vi "Meas Process Config Panel.vi"(8 "error in (no error)":errorcluster, 11 "session in":T1={"adc"={"niScope"={"channel cfg"=[], "sessions"=[], "multi cards"=FALSE, "channels"=0, "type"=enum."n/a", "memory [B/chn]"=0, "ext. clock [Hz]"=0.0, "samples count"=0, "use streaming"=FALSE, "proc setup"={"packet size [smpl]"=0, "current timeout [s]"=0.0, "blk2blk timeout [s]"=0.0, "event time"=timestamp(0 s since 1904-01-01), "temp sampl T [s]"=0.0, "data queue"=refnum, "stop notifier"=refnum, "proc ref"=refnum}, "sample width [B]"=0, "ranges [V]"=[], "trigger setup"={"coupling"=1, "level [V]"=0.0, "slope"=0, "mode"=enum."Immediate"}, "fs [Hz]"=0.0, "bitres [bit]"=0}, "3458A"={"channels"=[], "sync unit"={"VISA"="", "type"=enum."Picotest U6200A"}, "awg unit"={"type"=enum."Agilent 331xxA to 332xxA", "VISA"="", "enable 10MHz ref"=FALSE}, "sync mode"=enum."MASTER-SLAVE, MASTER clocked by TIMER", "streaming mode"=FALSE, "idn mode"=enum."Auto", "sampling mode"=enum."DCV", "Ts [s]"=0.0, "sample memory [B]"=0, "proc setup"={"channel id"=0, "packet size [smpl]"=0, "current timeout [s]"=0.0, "blk2blk timeout [s]"=0.0, "event time"=timestamp(0 s since 1904-01-01), "stop notifier"=refnum, "data queues"=[], "proc refs"=[], "bus semaphore"=refnum}, "sample size [B]"=0, "sample count"=0, "aux data"={"channel id"=0, "valid?"=[], "gain [V]"=[], "timestamp [s]"=[], "Ts [s]"=0.0, "abs timestamp"=timestamp(0 s since 1904-01-01), "t [deg C]"=[]}, "ranges [V]"=[], "aperture [s]"=0.0, "LEVEL trigger"={"edge"=enum."POS", "level [V]"=0.0, "coupling"=enum."DC"}, "trigger mode"=enum."AUTO", "measure temp.?"=FALSE, "disp mesages"=[], "shared bus?"=FALSE, "disable display?"=FALSE, "aper mode"=enum."Manual", "aper rules"=[]}, "dsdll"={"dsdll"={"dsdll path"=path "", "dsdll handle"=[], "output devices"=[], "capture devices"=[]}, "channels"=0, "device id"=0, "channel idns"=[], "proc setup"={"packet size [smpl]"=0, "current timeout [s]"=0.0, "blk2blk timeout [s]"=0.0, "event time"=timestamp(0 s since 1904-01-01), "data queue"=refnum, "stop notifier"=refnum, "proc ref"=refnum}, "samples count"=0, "fs [Hz]"=0.0}, "type"=enum."niScope", "channel idn str"=[], "aux instr idn str"=[], "modified?"=FALSE, "simadc"={"channels"=[], "range [V]"=0.0, "Ts step [s]"=0.0, "time [s]"=0.0, "fs [Hz]"=0.0, "count"=0, "smpl offset"=0, "set count"=0, "bit res"=0}, "force rst?"=FALSE, "exit mode"=enum."Immediate reset", "exit dly"=0.0, "exit tmr"=timestamp(0 s since 1904-01-01), "busy?"=FALSE, "accessed?"=FALSE, "QuADC session"={"channel cfg"=[], "sessions"=[], "multi cards"=FALSE, "channels"=0, "type"=enum."n/a", "memory [B/chn]"=0, "ext. clock [Hz]"=0.0, "samples count"=0, "use streaming"=FALSE, "proc setup"={"packet size [smpl]"=0, "current timeout [s]"=0.0, "blk2blk timeout [s]"=0.0, "event time"=timestamp(0 s since 1904-01-01), "temp sampl T [s]"=0.0, "data queue"=refnum, "stop notifier"=refnum, "proc ref"=refnum}, "sample width [B]"=0, "ranges [V]"=[], "trigger setup"={"coupling"=1, "level [V]"=0.0, "slope"=0, "mode"=enum."Immediate"}, "fs [Hz]"=0.0, "bitres [bit]"=0}}, "sequence"=[], "sequence setup"={"group setups"=[], "average cycles"=0, "range mode"=enum."Keep defaults", "fs mode"=enum."Frequency", "rng even"=0.0, "rng odd"=0.0, "folder"=path "", "name base"="", "meas id"=0, "settle [s]"=0.0}, "golpi"=refnum, "processing setup"={"mode"=enum."Raw", "call after avgs?"=FALSE, "calculate?"=FALSE, "raw mode"={"command"="", "result mode"=enum."Display console output (only Octave)", "res variable"=""}, "QWTB"={"QWTB path"=path "", "alg filter path"="", "alg ids"=[], "alg parameters"=[], "parsed parameters"=[], "selected alg id"="", "selected unc mode"=enum."None", "qwtb mcc"=100, "qwtb timeout"=90, "qwtb covg"=95.0, "qwtb ofs"=0, "qwtb lim data"=0, "multicore"={"jobs folder"=path "", "cores"=0, "max jobs"=0, "mode"=enum."Singlecore"}, "unc once?"=FALSE}}, "corrections"={"transducers"={"channels"=[], "last path"=path ""}, "digitizer"={"last path"=path "", "channel paths"=[], "channel idns"=[], "correction name"="", "channel names"=[], "folders to copy"=[], "channel valid"=[], "correction path"=path "", "correction rel path"="", "rel folders to copy"=[]}}, "assist cfg"={"P"=0, "Q"=0, "rel shift"=0.0, "ref freq"=0.0, "min fs"=0.0, "max fs tol"=0.0, "min int"=0.0, "max int"=0.0, "max err"=0.0, "max timeout"=0.0}} {"corrections"."transducers"."channels"."Phase index" min=1 step=1; "adc"."QuADC session"."trigger setup"."level [V]" format="%.2f"; "adc"."QuADC session"."trigger setup"."coupling" items=["AC"=0, "DC"=1, "HF Reject"=3, "LF Reject"=4, "AC Plus HF Reject"=1001]; "adc"."QuADC session"."channel cfg"."Clock fr. (Hz)" min=0.0 format="%#_9p"; "adc"."QuADC session"."channel cfg"."Number of JJ" min=1; "adc"."QuADC session"."channel cfg"."Range [Vpk]" min=0.0; "adc"."QuADC session"."channel cfg"."Channel" min=0; "adc"."3458A"."channels"."Range [Vpk]" min=0.0; "adc"."niScope"."trigger setup"."level [V]" format="%.2f"; "adc"."niScope"."trigger setup"."coupling" items=["AC"=0, "DC"=1, "HF Reject"=3, "LF Reject"=4, "AC Plus HF Reject"=1001]; "adc"."niScope"."channel cfg"."Range [Vpk]" min=0.0; "adc"."niScope"."channel cfg"."Channel" min=0}) -> (0 "error out":errorcluster, 3 "session out":T1={"adc"={"niScope"={"channel cfg"=[], "sessions"=[], "multi cards"=FALSE, "channels"=0, "type"=enum."n/a", "memory [B/chn]"=0, "ext. clock [Hz]"=0.0, "samples count"=0, "use streaming"=FALSE, "proc setup"={"packet size [smpl]"=0, "current timeout [s]"=0.0, "blk2blk timeout [s]"=0.0, "event time"=timestamp(0 s since 1904-01-01), "temp sampl T [s]"=0.0, "data queue"=refnum, "stop notifier"=refnum, "proc ref"=refnum}, "sample width [B]"=0, "ranges [V]"=[], "trigger setup"={"coupling"=1, "level [V]"=0.0, "slope"=0, "mode"=enum."Immediate"}, "fs [Hz]"=0.0, "bitres [bit]"=0}, "3458A"={"channels"=[], "sync unit"={"VISA"="", "type"=enum."Picotest U6200A"}, "awg unit"={"type"=enum."Agilent 331xxA to 332xxA", "VISA"="", "enable 10MHz ref"=FALSE}, "sync mode"=enum."MASTER-SLAVE, MASTER clocked by TIMER", "streaming mode"=FALSE, "idn mode"=enum."Auto", "sampling mode"=enum."DCV", "Ts [s]"=0.0, "sample memory [B]"=0, "proc setup"={"channel id"=0, "packet size [smpl]"=0, "current timeout [s]"=0.0, "blk2blk timeout [s]"=0.0, "event time"=timestamp(0 s since 1904-01-01), "stop notifier"=refnum, "data queues"=[], "proc refs"=[], "bus semaphore"=refnum}, "sample size [B]"=0, "sample count"=0, "aux data"={"channel id"=0, "valid?"=[], "gain [V]"=[], "timestamp [s]"=[], "Ts [s]"=0.0, "abs timestamp"=timestamp(0 s since 1904-01-01), "t [deg C]"=[]}, "ranges [V]"=[], "aperture [s]"=0.0, "LEVEL trigger"={"edge"=enum."POS", "level [V]"=0.0, "coupling"=enum."DC"}, "trigger mode"=enum."AUTO", "measure temp.?"=FALSE, "disp mesages"=[], "shared bus?"=FALSE, "disable display?"=FALSE, "aper mode"=enum."Manual", "aper rules"=[]}, "dsdll"={"dsdll"={"dsdll path"=path "", "dsdll handle"=[], "output devices"=[], "capture devices"=[]}, "channels"=0, "device id"=0, "channel idns"=[], "proc setup"={"packet size [smpl]"=0, "current timeout [s]"=0.0, "blk2blk timeout [s]"=0.0, "event time"=timestamp(0 s since 1904-01-01), "data queue"=refnum, "stop notifier"=refnum, "proc ref"=refnum}, "samples count"=0, "fs [Hz]"=0.0}, "type"=enum."niScope", "channel idn str"=[], "aux instr idn str"=[], "modified?"=FALSE, "simadc"={"channels"=[], "range [V]"=0.0, "Ts step [s]"=0.0, "time [s]"=0.0, "fs [Hz]"=0.0, "count"=0, "smpl offset"=0, "set count"=0, "bit res"=0}, "force rst?"=FALSE, "exit mode"=enum."Immediate reset", "exit dly"=0.0, "exit tmr"=timestamp(0 s since 1904-01-01), "busy?"=FALSE, "accessed?"=FALSE, "QuADC session"={"channel cfg"=[], "sessions"=[], "multi cards"=FALSE, "channels"=0, "type"=enum."n/a", "memory [B/chn]"=0, "ext. clock [Hz]"=0.0, "samples count"=0, "use streaming"=FALSE, "proc setup"={"packet size [smpl]"=0, "current timeout [s]"=0.0, "blk2blk timeout [s]"=0.0, "event time"=timestamp(0 s since 1904-01-01), "temp sampl T [s]"=0.0, "data queue"=refnum, "stop notifier"=refnum, "proc ref"=refnum}, "sample width [B]"=0, "ranges [V]"=[], "trigger setup"={"coupling"=1, "level [V]"=0.0, "slope"=0, "mode"=enum."Immediate"}, "fs [Hz]"=0.0, "bitres [bit]"=0}}, "sequence"=[], "sequence setup"={"group setups"=[], "average cycles"=0, "range mode"=enum."Keep defaults", "fs mode"=enum."Frequency", "rng even"=0.0, "rng odd"=0.0, "folder"=path "", "name base"="", "meas id"=0, "settle [s]"=0.0}, "golpi"=refnum, "processing setup"={"mode"=enum."Raw", "call after avgs?"=FALSE, "calculate?"=FALSE, "raw mode"={"command"="", "result mode"=enum."Display console output (only Octave)", "res variable"=""}, "QWTB"={"QWTB path"=path "", "alg filter path"="", "alg ids"=[], "alg parameters"=[], "parsed parameters"=[], "selected alg id"="", "selected unc mode"=enum."None", "qwtb mcc"=100, "qwtb timeout"=90, "qwtb covg"=95.0, "qwtb ofs"=0, "qwtb lim data"=0, "multicore"={"jobs folder"=path "", "cores"=0, "max jobs"=0, "mode"=enum."Singlecore"}, "unc once?"=FALSE}}, "corrections"={"transducers"={"channels"=[], "last path"=path ""}, "digitizer"={"last path"=path "", "channel paths"=[], "channel idns"=[], "correction name"="", "channel names"=[], "folders to copy"=[], "channel valid"=[], "correction path"=path "", "correction rel path"="", "rel folders to copy"=[]}}, "assist cfg"={"P"=0, "Q"=0, "rel shift"=0.0, "ref freq"=0.0, "min fs"=0.0, "max fs tol"=0.0, "min int"=0.0, "max int"=0.0, "max err"=0.0, "max timeout"=0.0}} {"corrections"."transducers"."channels"."Phase index" min=1 step=1; "adc"."QuADC session"."trigger setup"."level [V]" format="%.2f"; "adc"."QuADC session"."trigger setup"."coupling" items=["AC"=0, "DC"=1, "HF Reject"=3, "LF Reject"=4, "AC Plus HF Reject"=1001]; "adc"."QuADC session"."channel cfg"."Clock fr. (Hz)" min=0.0 format="%#_9p"; "adc"."QuADC session"."channel cfg"."Number of JJ" min=1; "adc"."QuADC session"."channel cfg"."Range [Vpk]" min=0.0; "adc"."QuADC session"."channel cfg"."Channel" min=0; "adc"."3458A"."channels"."Range [Vpk]" min=0.0; "adc"."niScope"."trigger setup"."level [V]" format="%.2f"; "adc"."niScope"."trigger setup"."coupling" items=["AC"=0, "DC"=1, "HF Reject"=3, "LF Reject"=4, "AC Plus HF Reject"=1001]; "adc"."niScope"."channel cfg"."Range [Vpk]" min=0.0; "adc"."niScope"."channel cfg"."Channel" min=0})   [LabVIEW 2013]
doc: "Configuration panel for result calculator. Select tab to select method of calculation."
uses:
  Meas Session.ctl
  adc/ADC Session.ctl
  drivers/niScope/niScope Session.ctl
  drivers/niScope/niScope Virtual Channel Config.ctl
  drivers/niScope/niScope Virtual Channel Mode.ctl
  drivers/niScope/niScope Virtual Channel Input Z.ctl
  drivers/niScope/niScope Virtual Channel Coupling.ctl
  drivers/niScope/niScope Type.ctl
  drivers/niScope/niScope Digitizing Process Options.ctl
  drivers/niScope/niScope Data Packet.ctl
  drivers/niScope/niScope Trigger Setup.ctl
  <instrlib>/niScope/Controls/niScope trigger coupling.ctl
  <instrlib>/niScope/Controls/niScope trigger slope.ctl
  drivers/DMM/3458A Digitizer Session.ctl
  drivers/DMM/3458A Virtual Channel Config.ctl
  drivers/Counter/Counter Session.ctl
  drivers/Counter/Counter Type.ctl
  drivers/AWG/AWG Session.ctl
  drivers/AWG/AWG Type.ctl
  drivers/DMM/3458A Sync Mode.ctl
  drivers/DMM/3458A Idn Mode.ctl
  drivers/DMM/3458A Digitizing Low Levels/Configure/Sampling Mode.ctl
  drivers/DMM/3458A Digitizing Process Options.ctl
  drivers/DMM/3458A Data Packet.ctl
  drivers/DMM/3458A Aux Record Data.ctl
  drivers/DMM/3458A Digitizing Low Levels/Configure/Level Setup.ctl
  drivers/DMM/3458A Digitizing Low Levels/Configure/First Sample Trigger.ctl
  drivers/DMM/3458A Aperture Selection Mode.ctl
  drivers/dsdll/DSDLL Session.ctl
  drivers/dsdll/dsdll.lvlibp/dsdll_instance.ctl
  drivers/dsdll/dsdll.lvlibp/dsdll_device_record.ctl
  drivers/dsdll/DSDLL Process Config.ctl
  drivers/dsdll/DSDLL Data Packet.ctl
  adc/ADC Type.ctl
  drivers/simulated_adc/SimAdc Config.ctl
  drivers/simulated_adc/SimAdc Channel Cfg.ctl
  adc/ADC On Close Action.ctl
  drivers/Quatsch_driver/QuADCDriver/QuADC Session.ctl
  drivers/Quatsch_driver/QuADCDriver/QuADC Virtual Channel Config.ctl
  drivers/Quatsch_driver/QuADCDriver/QuADC Virtual Channel Mode.ctl
  drivers/Quatsch_driver/QuADCDriver/QuADC Virtual Channel Input Z.ctl
  drivers/Quatsch_driver/QuADCDriver/QuADC Virtual Channel Coupling.ctl
  drivers/Quatsch_driver/QuADCDriver/QuADC Type.ctl
  drivers/Quatsch_driver/QuADCDriver/QuADC Digitizing Process Options.ctl
  drivers/Quatsch_driver/QuADCDriver/QuADC Data Packet.ctl
  drivers/Quatsch_driver/QuADCDriver/QuADC Trigger Setup.ctl
  Meas Sequence Item.ctl
  Meas Sampling Configuration.ctl
  adc/ADC Trig Config.ctl
  adc/ADC Trig Mode Source.ctl
  adc/ADC Trig Coupling.ctl
  adc/ADC Trig Slope.ctl
  QWTB/Meas Proc QWTB Algorithm Parameter Data.ctl
  Meas Sequence Configuration.ctl
  Meas Range Mode.ctl
  Meas Sampling Rate Mode.ctl
  octave/golpi/mpc/golpi_session_ref.ctl
  octave/golpi/mpc/golpi_session.ctl
  octave/golpi/GOLPI Library.lvlibp/Public/GOLPI reference Type Def.ctl
  octave/golpi/GOLPI Library.lvlibp/LV Process source distribution/Pipe Handle.ctl
  Meas Process Config.ctl
  Meas Process Mode.ctl
  Meas Process Raw Config.ctl
  Meas Process Raw Result Mode.ctl
  QWTB/Meas Proc QWTB Setup.ctl
  QWTB/Meas Proc QWTB Uncertainty Mode.ctl
  QWTB/Meas Proc QWTB Multicore Setup.ctl
  QWTB/Meas Proc QWTB Multicore Type.ctl
  Corrections/Corr Setup.ctl
  Corrections/Corr Tranducer Item.ctl
  Corrections/Corr Digitizers.ctl
  Assist/Assist Panel Setup.ctl
  varilib/SGUI Assign References Mode.ctl
  varilib/varilib.lvlib
  drivers/niScope/niScope Virtual Digitizer.lvlib
  drivers/DMM/3458A Virtual Digitizer.lvlib
  drivers/Counter/Counter.lvlib
  drivers/AWG/AWG.lvlib
  drivers/DMM/3458A Digitizing Low Levels/3458A Digitizing Low Levels.lvlib
  drivers/dsdll/dsdll.lvlibp
  drivers/dsdll/DSDLL Virtual Digitizer.lvlib
  octave/golpi/GOLPI Library.lvlibp/LV Process source distribution/LV Process library.lvlib
  octave/golpi/GOLPI Library.lvlibp
  octave/golpi/mpc/GOLPI Multi Process.lvlib
  drivers/Quatsch_driver/QuADCDriver/QuADC Virtual Digitizer.lvlib
panel:
  out "init parameters":bool=TRUE
  in  "btn fake":bool
  in  "btn ok":bool
  in  "tc mode":enum32{"RAW command", "QWTB"}(tab)
  in  "btn raw load m":bool
  in  "raw res var":string caption="Result string variable name"
  in  "raw res mode":T58 caption="Result display mode"
  in  "btn raw example":bool
  in  "raw calc once?":bool caption="Call just once when all averages are done?"
  in  "raw command":string="% load record sample data (path, group id, average id)\ndata = tpq_load_record(%header%, 0, %repid%);\n\n% calculate RMS (for coherent setup)\nrms = sum(data.y.^2,1).^0.5/data.sample_count^0.5\n\n% calculate DC offset (for coherent setup)\ndc = mean(data.y,1)\n\n% calculate spectrum\nN = size(data.y,1);\nU = fft(data.y)*2/N;\nU = U(1:floor(N/2),:)\nfs = [0:floor(N/2)-1]'/data.Ts/N;\n\n% plot it\nloglog(fs,abs(U));" caption="Octave/Matlab command string"
  in  "qwtb unc once":bool caption="Calculate uncertainty just once?"
  in  "qwtb lim data":bool caption="Limit input data:"
  in  "qwtb lim data size":i64 caption="Input data length [samples]"
  in  "qwtb data ofs":i64 caption="Start offset [sample]"
  in  "qwtb covg":dbl=95.0 caption="Level of Confidence [%]" min=50.0 max=99.99999
  in  "qwtb timeout":i32=90 caption="Processing timeout [s]"
  in  "qwtb mcc":i32=100 caption="Monte-Carlo cycles"
  out "qwtb alg has ui":bool caption="Algorithm expects two input (U and I)"
  out "qwtb alg is diff":bool caption="Algorithm supports differential transducer connection"
  in  "qwtb calc once":bool caption="Calculate result just once when\nall records are measured?"
  in  "qwtb unc mode":T60 caption="Uncertainty calculation mode"
  in  "btn qwtb clr params":bool
  out "qwtb var desc":string caption="Variable description"
  in  "qwtb alg params":string[][](table) caption="Parameters of the algorithm"
  out "qwtb alg cite":string caption="Citation"
  out "qwtb alg note":string caption="Note"
  out "qwtb alg desc":string caption="Description"
  in  "qwtb alg list":u16(ring) caption="List of algorithms" items=["SP-WFFT: Spectrum by means of Windowed Discrete Fourier Transform", "TWM-FPNLSF: TWM tool wrapper: Four Parameter Non-Linear Sine Fit", "TWM-Flicker: TWM tool wrapper: Flicker algorithm", "TWM-HCRMS: Half Cycle RMS algorithm", "TWM-InDiSwell: Interruption Dip Swell", "TWM-InpZ: TWM tool wrapper: Input impedance estimator", "TWM-MFSF: Multi Harmonic Frequency Estimator", "TWM-MODTDPS: TWM tool wrapper: Modulation estimator", "TWM-PSFE: TWM tool wrapper: Phase Sensitive Frequency Estimator", "TWM-PWRTDI: Power calculation algorithm using Time-Domain-Integration.", "TWM-PWRTEST: Test/demonstration algorithm for the TWM tool with two inputs", "TWM-TEST: Test/demonstration algorithm for the TWM tool", "TWM-THDWFFT: Harmonic distortion by windowed FFT", "TWM-WFFT: Windowed FFT for harmonic analysis.", "TWM-WRMS: RMS level calculation using windowed Time-Domain-Integration."]
  in  "btn load algs":bool
  in  "btn mc cfg":bool
  # "ADC:"
  # "IP Address"
  # "."
  # "."
  # "."
  # ":"
  # "ADC:"
  # "IP Address"
  # "."
  # "."
  # "."
  # ":"
  # "Enter Octave command sequence to execute. You can use following variables anywhere in the command sequence:\n\n%header% - full file path of the header file of the current measurement with no extension\n%repid% - id of the current repetition cycle (0 when calculating once after all repetitions are done)\n%respath% - result file path: '%header%-res.info' in the measurement folder"
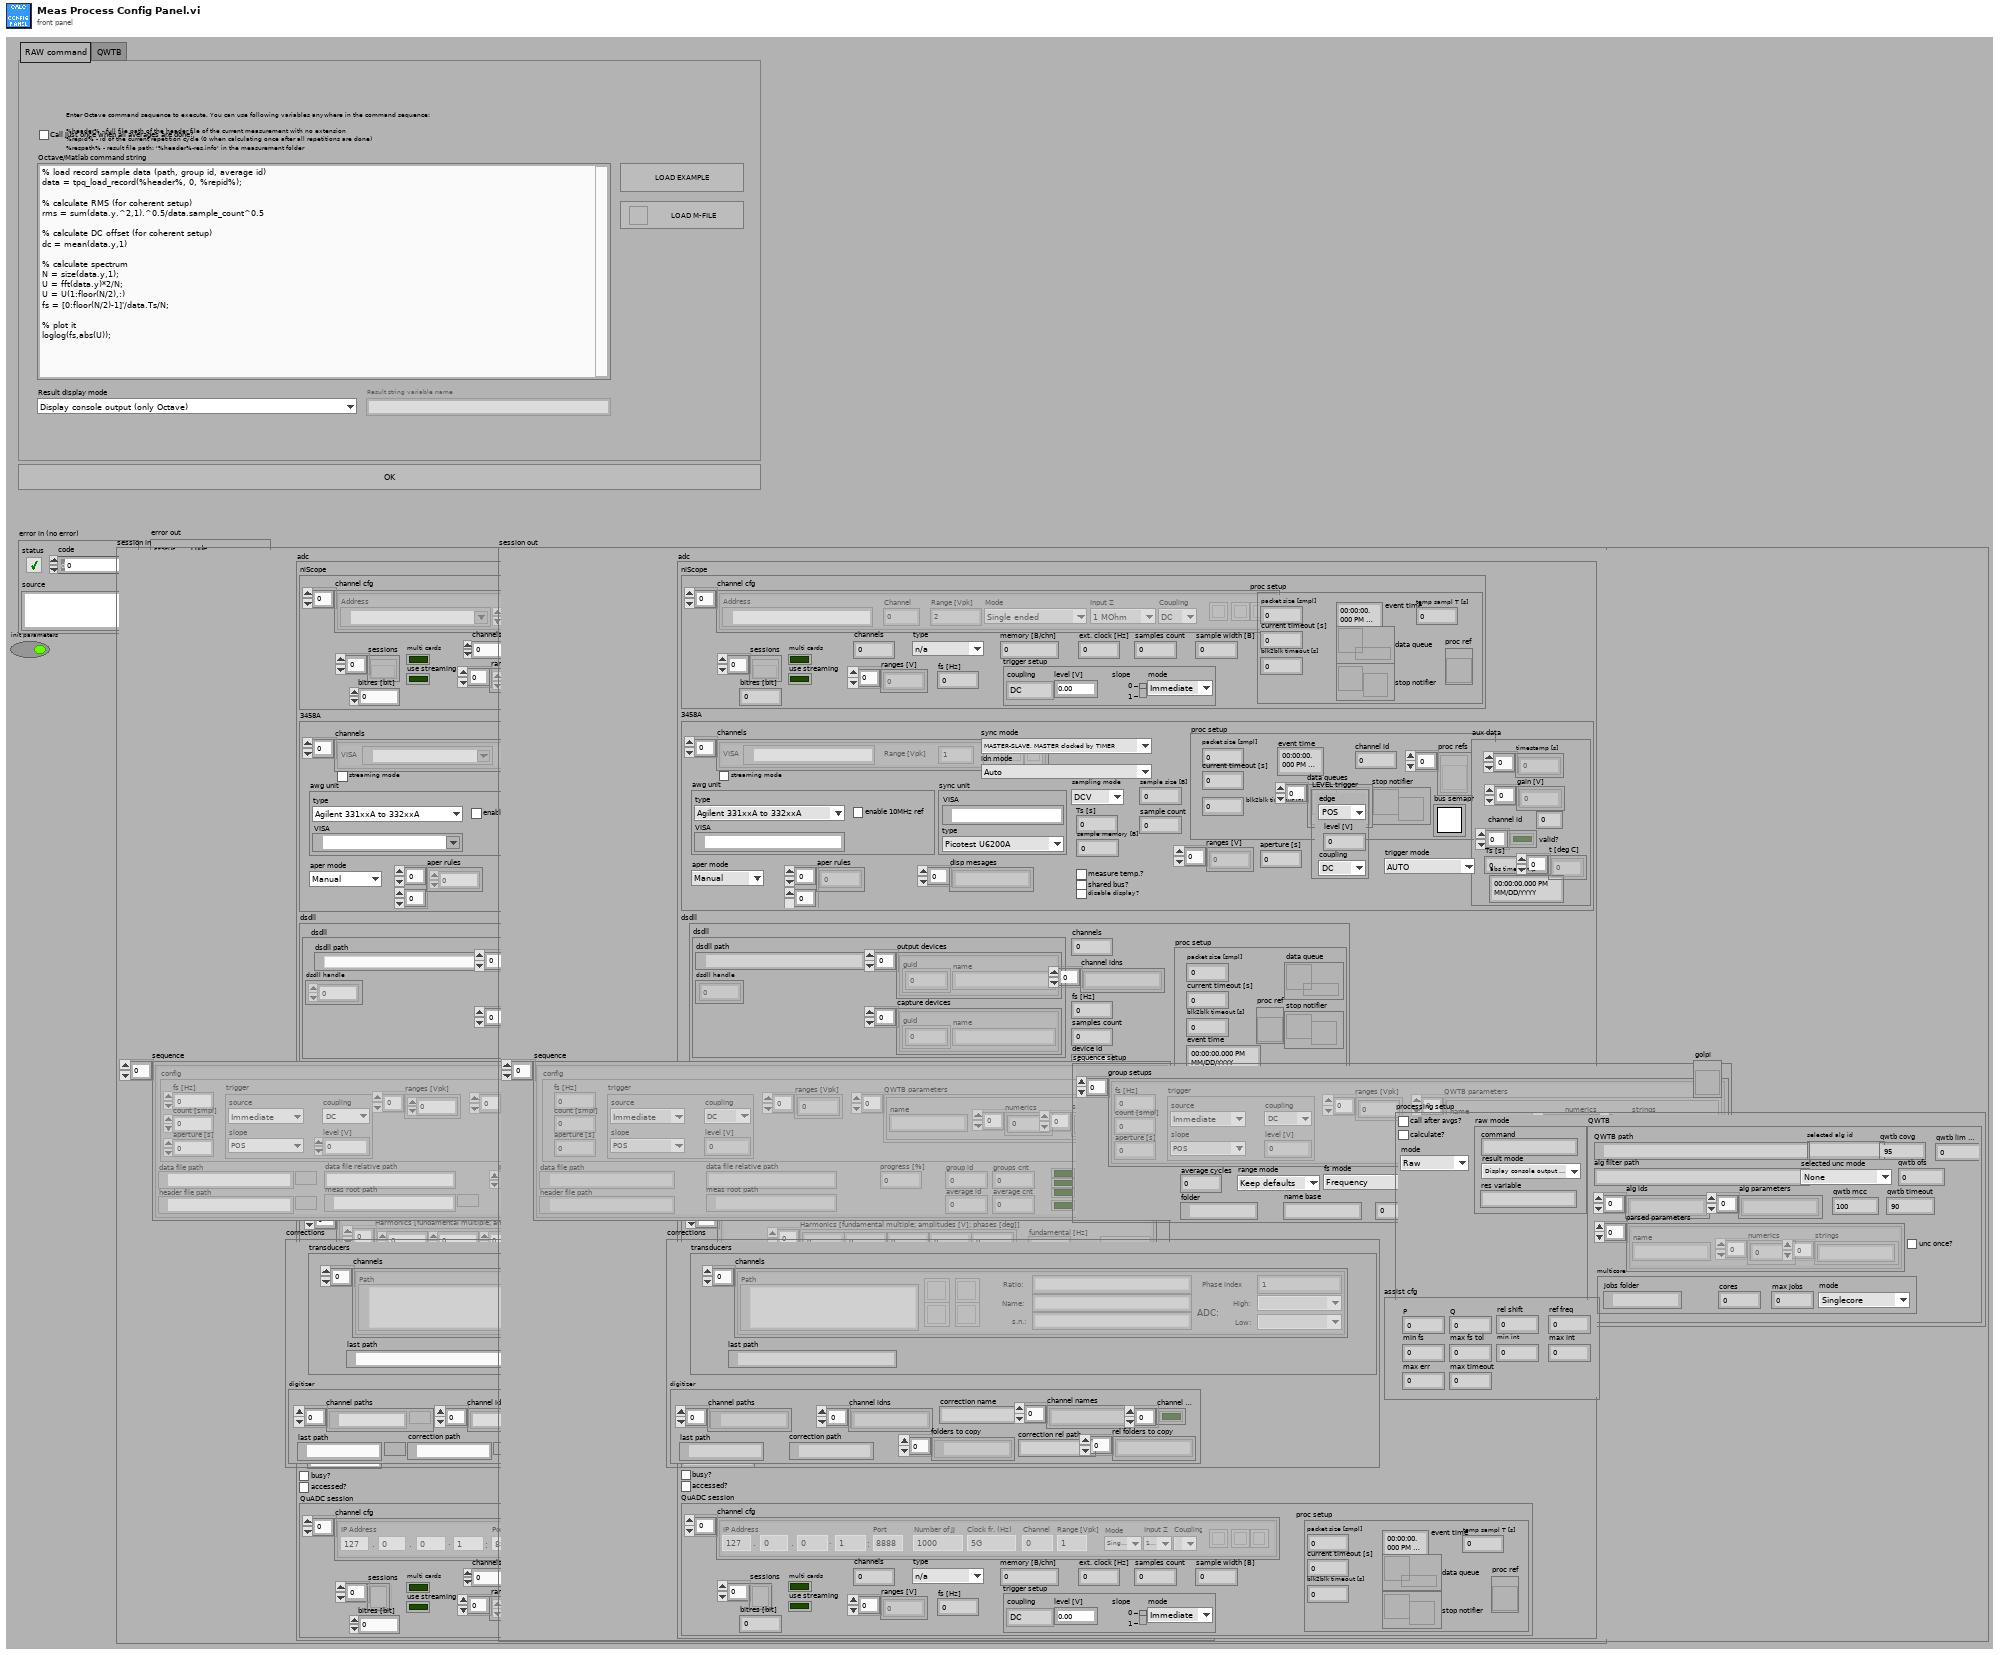
[diagram p1: front panel]
types:
  T1 = typedef "Meas Session.ctl" = cluster{"adc":T2, "sequence":T44[], "sequence setup":T51, "golpi":T54, "processing setup":T55, "corrections":T63, "assist cfg":T66}
  T2 = typedef "ADC Session.ctl" = cluster{"niScope":T3, "3458A":T13, "dsdll":T28, "type":T32, "channel idn str":string[], "aux instr idn str":string[], "modified?":bool, "simadc":T33, "force rst?":bool, "exit mode":T35, "exit dly":dbl, "exit tmr":timestamp, "busy?":bool, "accessed?":bool, "QuADC session":T36}
  T3 = typedef "niScope Virtual Digitizer.lvlib/niScope Session.ctl" = cluster{"channel cfg":T4[], "sessions":refnum<k20>[], "multi cards":bool, "channels":i32, "type":T8, "memory [B/chn]":i32, "ext. clock [Hz]":dbl, "samples count":i64, "use streaming":bool, "proc setup":T9, "sample width [B]":i32, "ranges [V]":dbl[], "trigger setup":T10, "fs [Hz]":dbl, "bitres [bit]":i32}
  T4 = typedef "niScope Virtual Digitizer.lvlib/niScope Virtual Channel Config.ctl" = cluster{"Address":refnum<k15>, "Channel":i32, "Mode":T5, "Input Z":T6, "Coupling":T7, "Range [Vpk]":dbl, "btn clr":bool, "btn up":bool, "btn down":bool}
  T5 = typedef "niScope Virtual Digitizer.lvlib/niScope Virtual Channel Mode.ctl" = enum16{"Single ended", "Unbal. differential", "Differential"}
  T6 = typedef "niScope Virtual Digitizer.lvlib/niScope Virtual Channel Input Z.ctl" = enum16{"1 MOhm", "50 Ohm"}
  T7 = typedef "niScope Virtual Digitizer.lvlib/niScope Virtual Channel Coupling.ctl" = enum16{"AC", "DC", "GND"}
  T8 = typedef "niScope Virtual Digitizer.lvlib/niScope Type.ctl" = enum16{"n/a", "5922"}
  T9 = typedef "niScope Virtual Digitizer.lvlib/niScope Digitizing Process Options.ctl" = cluster{"packet size [smpl]":i64, "current timeout [s]":dbl, "blk2blk timeout [s]":dbl, "event time":timestamp, "temp sampl T [s]":dbl, "data queue":refnum<queue>, "stop notifier":refnum<notifier>, "proc ref":refnum<vi>}
  T10 = typedef "niScope Virtual Digitizer.lvlib/niScope Trigger Setup.ctl" = cluster{"coupling":T11, "level [V]":dbl, "slope":T12, "mode":enum16{"Immediate", "External", "Level"}}
  T11 = typedef "niScope trigger coupling.ctl" = u16
  T12 = typedef "niScope trigger slope.ctl" = i32
  T13 = typedef "3458A Virtual Digitizer.lvlib/3458A Digitizer Session.ctl" = cluster{"channels":T14[], "sync unit":T15, "awg unit":T17, "sync mode":T19, "streaming mode":bool, "idn mode":T20, "sampling mode":T21, "Ts [s]":dbl, "sample memory [B]":i32, "proc setup":T22, "sample size [B]":i32, "sample count":i32, "aux data":T24, "ranges [V]":dbl[], "aperture [s]":dbl, "LEVEL trigger":T25, "trigger mode":T26, "measure temp.?":bool, "disp mesages":string[], "shared bus?":bool, "disable display?":bool, "aper mode":T27, "aper rules":dbl[][]}
  T14 = typedef "3458A Virtual Digitizer.lvlib/3458A Virtual Channel Config.ctl" = cluster{"VISA":refnum<visa-resource-name>, "Range [Vpk]":dbl, "btn clr":bool, "btn up":bool, "btn down":bool}
  T15 = typedef "Counter.lvlib/Counter Session.ctl" = cluster{"VISA":refnum<visa-resource-name>, "type":T16}
  T16 = typedef "Counter.lvlib/Counter Type.ctl" = enum16{"Picotest U6200A", "dummy"}
  T17 = typedef "AWG.lvlib/AWG Session.ctl" = cluster{"type":T18, "VISA":refnum<visa-resource-name>, "enable 10MHz ref":bool}
  T18 = typedef "AWG.lvlib/AWG Type.ctl" = enum16{"Agilent 331xxA to 332xxA", "Agilent 335xxA to 336xxA", "Tektronix AFG3101C", "dummy"}
  T19 = typedef "3458A Virtual Digitizer.lvlib/3458A Sync Mode.ctl" = enum16{"MASTER-SLAVE, MASTER clocked by TIMER", "MASTER-SLAVE, MASTER clocked by AWG", "ALL clocked by AWG", "MASTER-SLAVE, ALL clocked by TIMER", "ALL clocked by AWG with DFLL"}
  T20 = typedef "3458A Virtual Digitizer.lvlib/3458A Idn Mode.ctl" = enum16{"Auto", "Sequential (chn A, chn B, ...)", "From calibration string"}
  T21 = typedef "3458A Virtual Digitizer.lvlib/3458A Digitizing Low Levels.lvlib/Sampling Mode.ctl" = enum16{"DCV", "DSDC", "DSAC"}
  T22 = typedef "3458A Virtual Digitizer.lvlib/3458A Digitizing Process Options.ctl" = cluster{"channel id":i32, "packet size [smpl]":i32, "current timeout [s]":dbl, "blk2blk timeout [s]":dbl, "event time":timestamp, "stop notifier":refnum<notifier>, "data queues":refnum<queue>[], "proc refs":refnum<vi>[], "bus semaphore":T23}
  T23 = typedef "Semaphore RefNum" = refnum<k1>
  T24 = typedef "3458A Virtual Digitizer.lvlib/3458A Aux Record Data.ctl" = cluster{"channel id":i32, "valid?":bool[], "gain [V]":dbl[], "timestamp [s]":dbl[], "Ts [s]":dbl, "abs timestamp":timestamp, "t [deg C]":dbl[]}
  T25 = typedef "3458A Virtual Digitizer.lvlib/3458A Digitizing Low Levels.lvlib/Level Setup.ctl" = cluster{"edge":enum16{"POS", "NEG"}, "level [V]":dbl, "coupling":enum16{"DC", "AC"}}
  T26 = typedef "3458A Virtual Digitizer.lvlib/3458A Digitizing Low Levels.lvlib/First Sample Trigger.ctl" = enum16{"AUTO", "EXT", "SYN", "SGL", "HOLD", "LEVEL"}
  T27 = typedef "3458A Virtual Digitizer.lvlib/3458A Aperture Selection Mode.ctl" = enum16{"Manual", "Maximum", "Table"}
  T28 = typedef "DSDLL Virtual Digitizer.lvlib/DSDLL Session.ctl" = cluster{"dsdll":T29, "channels":i32, "device id":i32, "channel idns":string[], "proc setup":T31, "samples count":i32, "fs [Hz]":dbl}
  T29 = typedef "dsdll.lvlibp/dsdll_instance.ctl" = cluster{"dsdll path":path, "dsdll handle":u8[], "output devices":T30[], "capture devices":T30[]}
  T30 = typedef "dsdll.lvlibp/dsdll_device_record.ctl" = cluster{"guid":u8[], "name":string}
  T31 = typedef "DSDLL Virtual Digitizer.lvlib/DSDLL Process Config.ctl" = cluster{"packet size [smpl]":i32, "current timeout [s]":dbl, "blk2blk timeout [s]":dbl, "event time":timestamp, "data queue":refnum<queue>, "stop notifier":refnum<notifier>, "proc ref":refnum<vi>}
  T32 = typedef "ADC Type.ctl" = enum16{"niScope", "3458A", "DirectSound DLL", "dummy", "QuADC"}
  T33 = typedef "SimAdc Config.ctl" = cluster{"channels":T34[], "range [V]":dbl, "Ts step [s]":dbl, "time [s]":dbl, "fs [Hz]":dbl, "count":i64, "smpl offset":i64, "set count":i64, "bit res":i32}
  T34 = typedef "SimAdc Channel Cfg.ctl" = cluster{"harmonics":dbl[][], "btn clear":bool, "noise":dbl, "fundamental [Hz]":dbl}
  T35 = typedef "ADC On Close Action.ctl" = enum16{"Immediate reset", "Delayed reset"}
  T36 = typedef "QuADC Virtual Digitizer.lvlib/QuADC Session.ctl" = cluster{"channel cfg":T37[], "sessions":refnum<k5>[], "multi cards":bool, "channels":i32, "type":T41, "memory [B/chn]":i32, "ext. clock [Hz]":dbl, "samples count":i64, "use streaming":bool, "proc setup":T42, "sample width [B]":i32, "ranges [V]":dbl[], "trigger setup":T43, "fs [Hz]":dbl, "bitres [bit]":i32}
  T37 = typedef "QuADC Virtual Digitizer.lvlib/QuADC Virtual Channel Config.ctl" = cluster{"Channel":i32, "Mode":T38, "Input Z":T39, "Coupling":T40, "Range [Vpk]":dbl, "btn clr":bool, "btn up":bool, "btn down":bool, "IP address A":u8, "IP address B":u8, "IP address C":u8, "IP address D":u8, "Port":u16, "Number of JJ":u32, "Clock fr. (Hz)":dbl}
  T38 = typedef "QuADC Virtual Digitizer.lvlib/QuADC Virtual Channel Mode.ctl" = enum16{"Single ended", "Unbal. differential", "Differential"}
  T39 = typedef "QuADC Virtual Digitizer.lvlib/QuADC Virtual Channel Input Z.ctl" = enum16{"1 MOhm", "50 Ohm"}
  T40 = typedef "QuADC Virtual Digitizer.lvlib/QuADC Virtual Channel Coupling.ctl" = enum16{"AC", "DC", "GND"}
  T41 = typedef "QuADC Virtual Digitizer.lvlib/QuADC Type.ctl" = enum16{"n/a", "v1"}
  T42 = typedef "QuADC Virtual Digitizer.lvlib/QuADC Digitizing Process Options.ctl" = cluster{"packet size [smpl]":i64, "current timeout [s]":dbl, "blk2blk timeout [s]":dbl, "event time":timestamp, "temp sampl T [s]":dbl, "data queue":refnum<queue>, "stop notifier":refnum<notifier>, "proc ref":refnum<vi>}
  T43 = typedef "QuADC Virtual Digitizer.lvlib/QuADC Trigger Setup.ctl" = cluster{"coupling":T11, "level [V]":dbl, "slope":T12, "mode":enum16{"Immediate", "External", "Level"}}
  T44 = typedef "Meas Sequence Item.ctl" = cluster{"config":T45, "data file path":path, "header file path":path, "group id":i32, "average id":i32, "group done?":bool, "adc modified?":bool, "source modified?":bool, "progress [%]":dbl, "groups cnt":i32, "average cnt":i32, "data file relative path":string, "meas root path":path, "calculate?":bool}
  T45 = typedef "Meas Sampling Configuration.ctl" = cluster{"fs [Hz]":dbl, "count [smpl]":i64, "aperture [s]":dbl, "trigger":T46, "ranges [Vpk]":dbl[], "QWTB parameters":T50[]}
  T46 = typedef "ADC Trig Config.ctl" = cluster{"source":T47, "level [V]":dbl, "coupling":T48, "slope":T49}
  T47 = typedef "ADC Trig Mode Source.ctl" = enum16{"Immediate", "External", "Level"}
  T48 = typedef "ADC Trig Coupling.ctl" = enum16{"DC", "AC"}
  T49 = typedef "ADC Trig Slope.ctl" = enum16{"POS", "NEG"}
  T50 = typedef "Meas Proc QWTB Algorithm Parameter Data.ctl" = cluster{"name":string, "numerics":dbl[], "strings":string[]}
  T51 = typedef "Meas Sequence Configuration.ctl" = cluster{"group setups":T45[], "average cycles":i32, "range mode":T52, "fs mode":T53, "rng even":dbl, "rng odd":dbl, "folder":path, "name base":string, "meas id":i32, "settle [s]":dbl}
  T52 = typedef "Meas Range Mode.ctl" = enum16{"Keep defaults", "Set All channels", "Set Odd and Even channels"}
  T53 = typedef "Meas Sampling Rate Mode.ctl" = enum16{"Frequency", "Period"}
  T54 = typedef "GOLPI Multi Process.lvlib/golpi_session_ref.ctl" = refnum<vi>
  T55 = typedef "Meas Process Config.ctl" = cluster{"mode":T56, "call after avgs?":bool, "calculate?":bool, "raw mode":T57, "QWTB":T59}
  T56 = typedef "Meas Process Mode.ctl" = enum16{"Raw", "QWTB"}
  T57 = typedef "Meas Process Raw Config.ctl" = cluster{"command":string, "result mode":T58, "res variable":string}
  T58 = typedef "Meas Process Raw Result Mode.ctl" = enum16{"Display console output (only Octave)", "Display string variable", "Display result file %respath%"}
  T59 = typedef "Meas Proc QWTB Setup.ctl" = cluster{"QWTB path":path, "alg filter path":string, "alg ids":string[], "alg parameters":string[], "parsed parameters":T50[], "selected alg id":string, "selected unc mode":T60, "qwtb mcc":i32, "qwtb timeout":i32, "qwtb covg":dbl, "qwtb ofs":i64, "qwtb lim data":i64, "multicore":T61, "unc once?":bool}
  T60 = typedef "Meas Proc QWTB Uncertainty Mode.ctl" = enum16{"None", "GUF", "Monte Carlo"}
  T61 = typedef "Meas Proc QWTB Multicore Setup.ctl" = cluster{"jobs folder":path, "cores":i32, "max jobs":i32, "mode":T62}
  T62 = typedef "Meas Proc QWTB Multicore Type.ctl" = enum16{"Singlecore", "Multicore", "Multistation"}
  T63 = typedef "Corr Setup.ctl" = cluster{"transducers":cluster{"channels":T64[], "last path":path}, "digitizer":T65}
  T64 = typedef "Corr Tranducer Item.ctl" = cluster{"Path":path, "Ratio:":string, "Name:":string, "btn rem":bool, "btn up":bool, "btn down":bool, "s.n.:":string, "btn open":bool, "ratio o/i":dbl, "chn hi":u16, "chn lo":u16, "Phase index":i32}
  T65 = typedef "Corr Digitizers.ctl" = cluster{"last path":path, "channel paths":path[], "channel idns":string[], "correction name":string, "channel names":string[], "folders to copy":path[], "channel valid":bool[], "correction path":path, "correction rel path":string, "rel folders to copy":string[]}
  T66 = typedef "Assist Panel Setup.ctl" = cluster{"P":i32, "Q":i32, "rel shift":dbl, "ref freq":dbl, "min fs":dbl, "max fs tol":dbl, "min int":dbl, "max int":dbl, "max err":dbl, "max timeout":dbl}
  T67 = typedef "varilib.lvlib/SGUI Assign References Mode.ctl" = enum16{"Add to stack", "Overwrite", "Release last", "Release ID"}
  T68 = typedef "Meas Proc QWTB Algorithm Flags.ctl" = cluster{"supports multiple records?":bool, "supports differential transducer?":bool, "dual input algorithm?":bool}
  T69 = typedef "Meas Proc QWTB Algorithm Info.ctl" = cluster{"name":string, "description":string, "citation":string, "remark":string, "license":string}
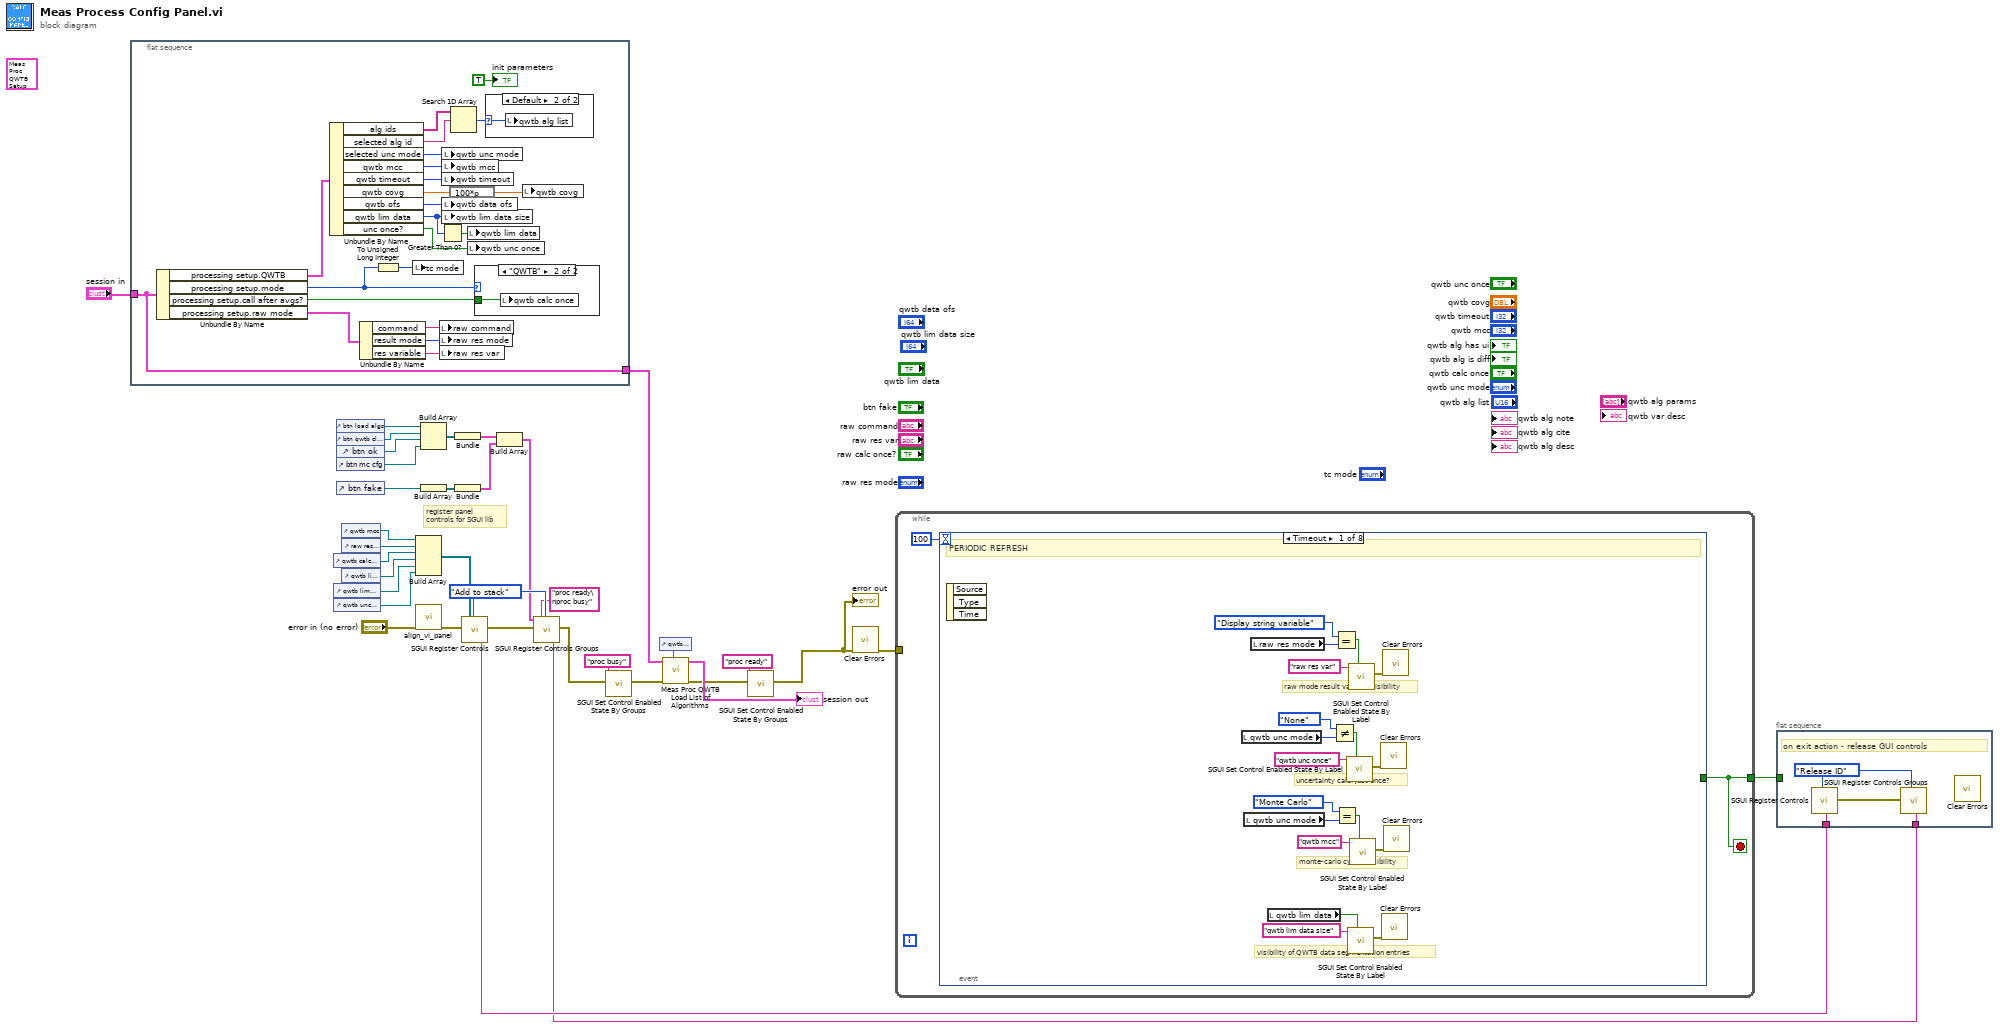
[diagram p0: block diagram]
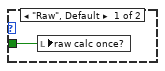
[diagram p3: hidden frame]
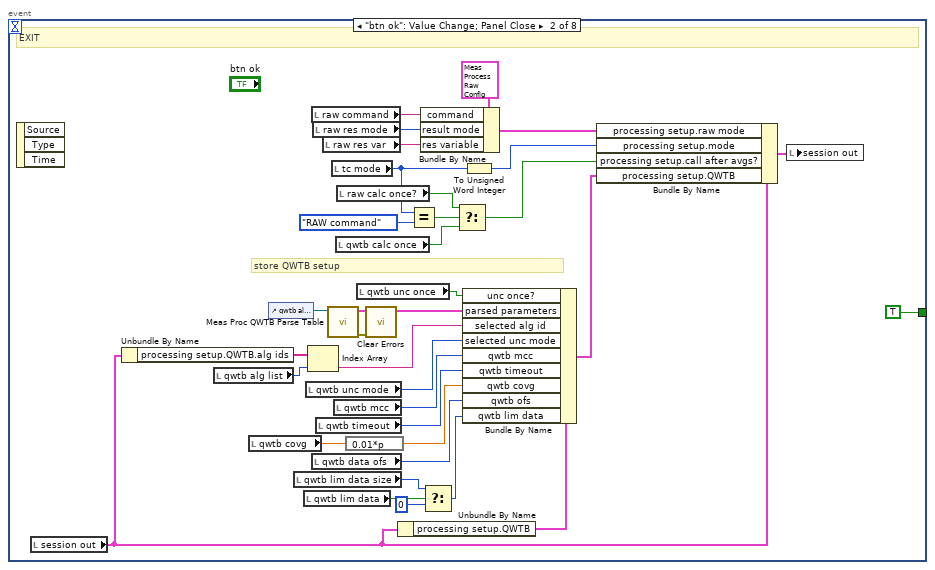
[diagram p4: hidden frame]
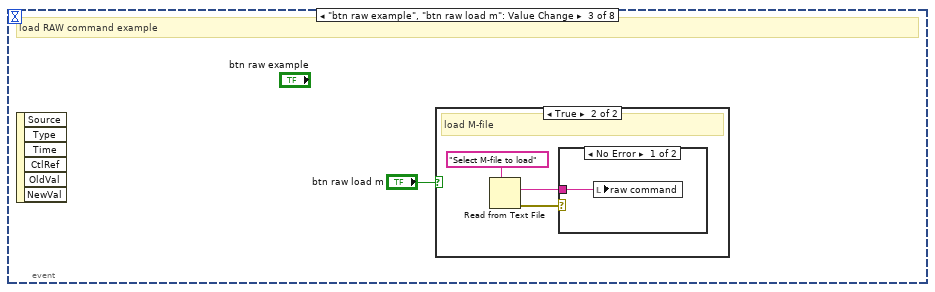
[diagram p5: hidden frame]
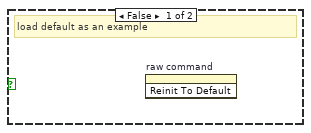
[diagram p6: hidden frame]
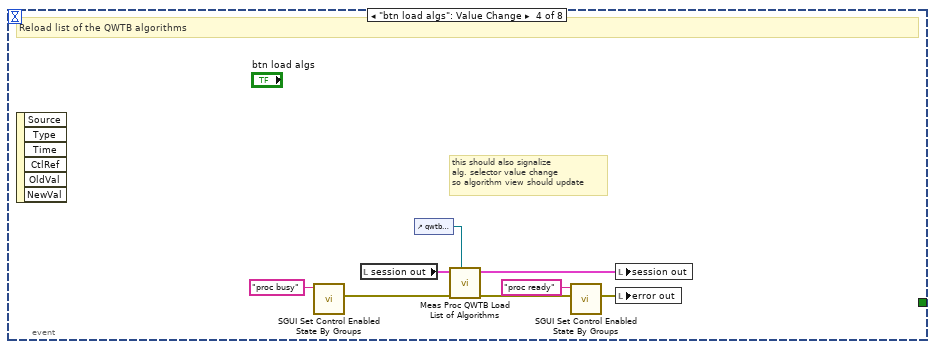
[diagram p8: hidden frame]
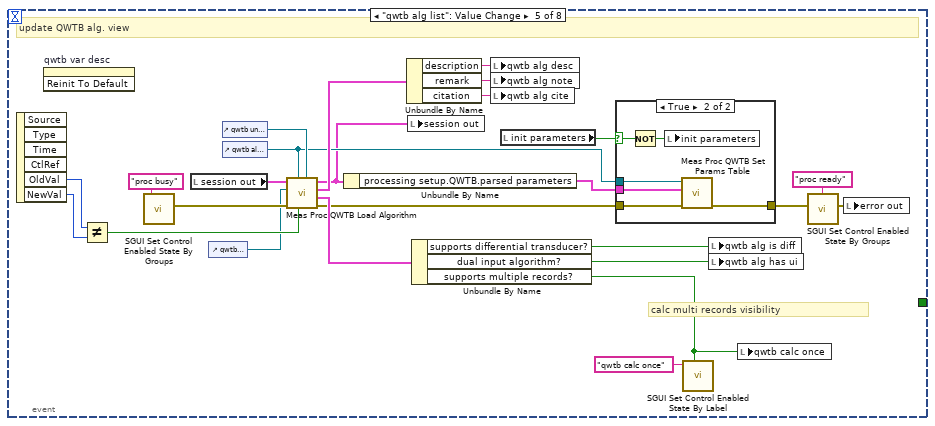
[diagram p9: hidden frame]
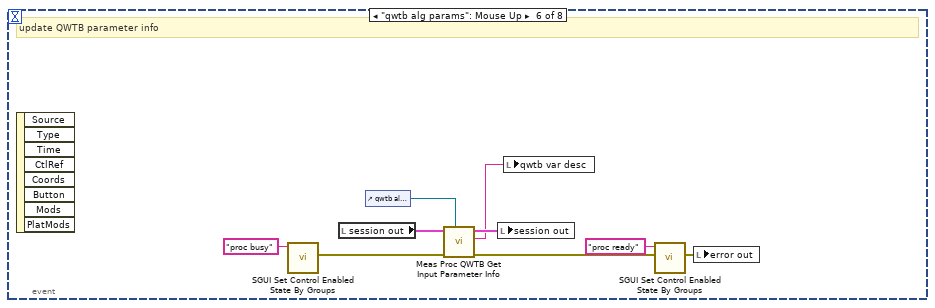
[diagram p11: hidden frame]
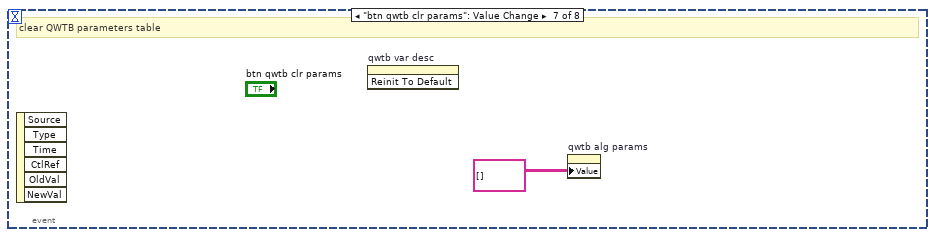
[diagram p12: hidden frame]
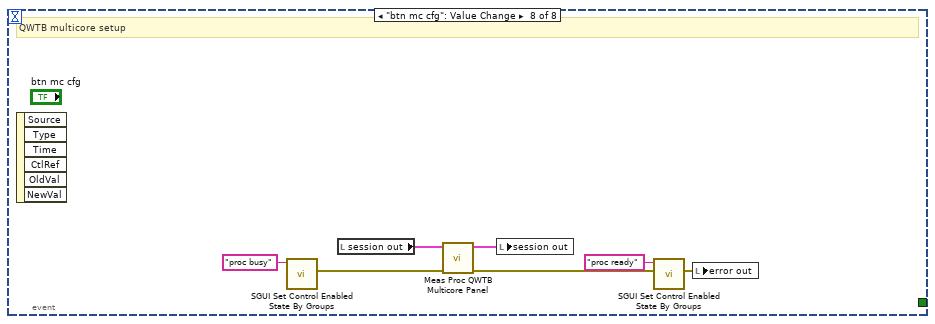
[diagram p13: hidden frame]
diagram:
  (unwired) T59 {"QWTB path"=path "", "alg filter path"="", "alg ids"=[], "alg parameters"=[], "parsed parameters"=[], "selected alg id"="", "selected unc mode"=enum."None", "qwtb mcc"=0, "qwtb timeout"=0, "qwtb covg"=0.0, "qwtb ofs"=0, "qwtb lim data"=0, "multicore"={"jobs folder"=path "", "cores"=0, "max jobs"=0, "mode"=enum."Singlecore"}, "unc once?"=FALSE} ("processing setup.QWTB")
  w23 = SGUI_Assign_References_Mode."Add to stack" ("register mode (overwrite)")
  # "register panel\ncontrols for SGUI lib"
  n1 = flat-sequence {
    tunnel: "session in" -> [w49]
    tunnel: [w49] -> w28
    frame #0 {
      n2 = Unbundle By Name(w49) -> ("processing setup.QWTB"=w51:T59, "processing setup.mode"=w53:T56, "processing setup.call after avgs?"=w52:bool, "processing setup.raw mode"=w57:T57)
      n3 = Unbundle By Name(w51) -> ("alg ids"=w44:string[], "selected alg id"=w43:string, "selected unc mode"=w50:T60, "qwtb mcc"=w48:i32, "qwtb timeout"=w47:i32, "qwtb covg"=w46:dbl, "qwtb ofs"=w40:i64, "qwtb lim data"=w38:i64, "unc once?"=w37:bool)
      n4 = Unbundle By Name(w57) -> ("command"=w56:string, "result mode"=w55:T58, "res variable"=w54:string)
      n5 = To Unsigned Long Integer(number=w53) -> (unsigned 32bit integer=w58:u32)
      n6 = local write "tc mode"(w58) -> ()
      n7 = Greater Than 0?(x=w38) -> (x > 0?=w39:bool)
      n8 = local write "raw command"(w56) -> ()
      n9 = local write "raw res mode"(w55) -> ()
      n10 = local write "raw res var"(w54) -> ()
      n11 = local write "qwtb unc mode"(w50) -> ()
      n12 = local write "qwtb mcc"(w48) -> ()
      n13 = local write "qwtb timeout"(w47) -> ()
      n14 = local write "qwtb data ofs"(w40) -> ()
      n15 = local write "qwtb lim data size"(w38) -> ()
      n16 = expression code="100*p"(w46) -> (w45:dbl)
      n17 = Search 1D Array(1D array=w44, element=w43) -> (index of element=w42:i32)  [unwired: 1 in]
      n18 = local write "qwtb lim data"(w39) -> ()
      n19 = local write "qwtb unc once"(w37) -> ()
      n20 = case shown="\"QWTB\"" w53 {
        tunnel: w52 -> [w60 w61]
        frame "Raw", Default {
          n21 = local write "raw calc once?"(w60) -> ()
        }
        frame "QWTB" {
          n22 = local write "qwtb calc once"(w61) -> ()
        }
      }
      n23 = case shown="Default" w42 {
        selector: w42 -> [_ w59]
        frame -1 {
        }
        frame Default {
          n24 = local write "qwtb alg list"(w59) -> ()
        }
      }
      n25 = local write "qwtb covg"(w45) -> ()
      "init parameters" <- TRUE ("init parameters")
    }
  }
  n26 = control-ref of="qwtb calc once"() -> (w27:refnum<vi>)
  n27 = control-ref of="qwtb lim data"() -> (w3:refnum<vi>)
  n28 = control-ref of="qwtb unc once"() -> (w1:refnum<vi>)
  n29 = control-ref of="btn load algs"() -> (w15:refnum<vi>)
  n30 = control-ref of="btn qwtb clr params"() -> (w14:refnum<vi>)
  n31 = control-ref of="btn ok"() -> (w13:refnum<vi>)
  n32 = control-ref of="btn mc cfg"() -> (w2:refnum<vi>)
  n33 = control-ref of="btn fake"() -> (w12:refnum<vi>)
  n34 = control-ref of="qwtb mcc"() -> (w26:refnum<vi>)
  n35 = control-ref of="raw res var"() -> (w35:refnum<vi>)
  n36 = control-ref of="qwtb lim data size"() -> (w4:refnum<vi>)
  n37 = Build Array(w26, w35, w27, w4, w3, w1) -> (w36:refnum<vi>[])
  n38 = call "align_vi_panel.vi"("error in"="error in (no error)") -> ("error out"=w32:errorcluster)  [unwired: 10 in]
  n39 = Build Array(w15, w14, w13, w2) -> (w21:refnum<vi>[])
  n40 = Build Array(w12) -> (w19:refnum<vi>[])
  n41 = Bundle(w21) -> (w22:cluster{refnum<vi>[]})  [unwired: 1 in]
  n42 = Bundle(w19) -> (w20:cluster{refnum<vi>[]})  [unwired: 1 in]
  n43 = call "SGUI Register Controls.vi"("error in"=w32, "control references (empty)"=w36, "register mode (overwrite)"=w23) -> ("assigned ID"=w25:string, "error out"=w24:errorcluster)  [unwired: 14 in, 1 out]
  n44 = Build Array(w22, w20) -> (w17:cluster{refnum<vi>[]}[])
  n45 = call "SGUI Register Controls Groups.vi"("control groups"=w17, "error in"=w24, "groups names"="proc ready\nproc busy", "register mode (overwrite)"=w23) -> ("assigned ID"=w16:string, "error out"=w8:errorcluster)  [unwired: 14 in]
  n46 = call "SGUI Set Control Enabled State By Groups.vi"("error in"=w8, "group name to enable (none)"="proc busy") -> ("error out"=w9:errorcluster)  [unwired: 8 in, 1 out]
  n47 = control-ref of="qwtb alg list"() -> (w29:refnum<vi>)
  n48 = call "Meas Proc QWTB Load List of Algorithms.vi"("menu ring ref"=w29, "error in"=w9, "session in"=w28) -> ("error out"=w6:errorcluster, "session out"=→"session out":T1)  [unwired: 6 in, 1 out]
  n49 = call "SGUI Set Control Enabled State By Groups.vi"("error in"=w6, "group name to enable (none)"="proc ready") -> ("error out"=w5:errorcluster)  [unwired: 8 in, 1 out]
  "error out" <- w5
  n50 = call <vilib>:"Clear Errors.vi"("error in (no error)"=w5) -> ("error out"=w34:errorcluster)  [unwired: 6 in]
  n51 = while {
    tunnel: w34 -> [_]
    tunnel: [w62] -> w33
    stop <- w62 stop-if-true
    n52 = event shown="[0] Timeout" {
      selector: _ -> [_ _ _ _ _ _ _ _]
      dyn-events: _ -> [_ _ _ _ _ _ _ _]
      timeout: 100 -> [_ _ _ _ _ _ _ _]
      tunnel: [_ TRUE _ _ _ _ _ _] -> w62
      event Timeout {
        # "uncertainty calc. just once?"
        # "visibility of QWTB data segmentation entries"
        # "monte-carlo cycles visibility"
        # "raw mode result variable visibility"
        # "PERIODIC REFRESH"
        n53 = event-data() -> ()  [unwired: 1 in, 3 out]
        n54 = local read "qwtb unc mode"() -> (w67:T60)
        n55 = local read "qwtb unc mode"() -> (w73:T60)
        n56 = local read "raw res mode"() -> (w81:T58)
        n57 = local read "qwtb lim data"() -> (w71:bool)
        n58 = Not Equal?(x=Meas_Proc_QWTB_Uncertainty_Mode."None", y=w67) -> (x != y?=w66:bool)
        n59 = Equal?(x=Meas_Process_Raw_Result_Mode."Display string variable", y=w81) -> (x = y?=w79:bool)
        n60 = Equal?(x=Meas_Proc_QWTB_Uncertainty_Mode."Monte Carlo", y=w73) -> (x = y?=w74:bool)
        n61 = call "SGUI Set Control Enabled State By Label.vi"("labels (empty)"="qwtb unc once", "Enabled? (False)"=w66) -> ("error out"=w64:errorcluster)  [unwired: 8 in, 1 out]
        n62 = call "SGUI Set Control Enabled State By Label.vi"("labels (empty)"="qwtb lim data size", "Enabled? (False)"=w71) -> ("error out"=w69:errorcluster)  [unwired: 8 in, 1 out]
        n63 = call "SGUI Set Control Enabled State By Label.vi"("labels (empty)"="raw res var", "Enabled? (False)"=w79) -> ("error out"=w77:errorcluster)  [unwired: 8 in, 1 out]
        n64 = call "SGUI Set Control Enabled State By Label.vi"("labels (empty)"="qwtb mcc", "Enabled? (False)"=w74) -> ("error out"=w76:errorcluster)  [unwired: 8 in, 1 out]
        n65 = call <vilib>:"Clear Errors.vi"("error in (no error)"=w64) -> ()  [unwired: 6 in, 1 out]
        n66 = call <vilib>:"Clear Errors.vi"("error in (no error)"=w69) -> ()  [unwired: 6 in, 1 out]
        n67 = call <vilib>:"Clear Errors.vi"("error in (no error)"=w77) -> ()  [unwired: 6 in, 1 out]
        n68 = call <vilib>:"Clear Errors.vi"("error in (no error)"=w76) -> ()  [unwired: 6 in, 1 out]
      }
      event "btn ok": Value Change; Panel Close {
        # "store QWTB setup"
        # "EXIT"
        n69 = event-data() -> ()  [unwired: 1 in, 3 out]
        n70 = local read "session out"() -> (w91:T1)
        n71 = Unbundle By Name(w91) -> ("processing setup.QWTB.alg ids"=w90:string[])
        n72 = local read "qwtb alg list"() -> (w89:u16)
        n73 = local read "qwtb covg"() -> (w93:dbl)
        n74 = control-ref of="qwtb alg params"() -> (w101:refnum<vi>)
        n75 = local read "qwtb lim data size"() -> (w84:i64)
        n76 = local read "qwtb lim data"() -> (w86:bool)
        n77 = local read "qwtb unc mode"() -> (w99:T60)
        n78 = Index Array(array=w90, index=w89) -> (element=w88:string)
        n79 = local read "raw command"() -> (w114:string)
        n80 = local read "qwtb data ofs"() -> (w87:i64)
        n81 = local read "raw res mode"() -> (w113:T58)
        n82 = local read "qwtb timeout"() -> (w94:i32)
        n83 = local read "raw res var"() -> (w112:string)
        n84 = call "Meas Proc QWTB Parse Table.vi"("param table ref"=w101) -> ("error out"=w100:errorcluster, "qwtb parameters"=w102:T50[])  [unwired: 9 in]
        n85 = local read "tc mode"() -> (w104:enum32{"RAW command", "QWTB"})
        n86 = local read "qwtb mcc"() -> (w95:i32)
        n87 = local read "qwtb calc once"() -> (w97:bool)
        n88 = local read "raw calc once?"() -> (w108:bool)
        n89 = expression code="0.01*p"(w93) -> (w92:dbl)
        n90 = local read "qwtb unc once"() -> (w82:bool)
        n91 = call <vilib>:"Clear Errors.vi"("error in (no error)"=w100) -> ()  [unwired: 6 in, 1 out]
        n92 = Unbundle By Name(w91) -> ("processing setup.QWTB"=w96:T59)
        n93 = Equal?(x=w104, y=enum32{"RAW command", "QWTB"}."RAW command") -> (x = y?=w109:bool)
        n94 = Bundle By Name(cluster=T57 {"command"="", "result mode"=enum."Display result file %respath%", "res variable"=""} ("raw mode"), "command"=w114, "result mode"=w113, "res variable"=w112) -> (w111:T57)
        n95 = Select(t=w84, s=w86, f=i64 0) -> (s? t:f=w85:i64)
        n96 = Select(t=w108, s=w109, f=w97) -> (s? t:f=w107:bool)
        n97 = Bundle By Name(cluster=w96, "unc once?"=w82, "parsed parameters"=w102, "selected alg id"=w88, "selected unc mode"=w99, "qwtb mcc"=w95, "qwtb timeout"=w94, "qwtb covg"=w92, "qwtb ofs"=w87, "qwtb lim data"=w85) -> (w98:T59)
        n98 = To Unsigned Word Integer(number=w104) -> (unsigned 16bit integer=w103:u16)
        n99 = Bundle By Name(cluster=w91, "processing setup.raw mode"=w111, "processing setup.mode"=w103, "processing setup.call after avgs?"=w107, "processing setup.QWTB"=w98) -> (w106:T1)
        n100 = local write "session out"(w106) -> ()
      }
      event "btn raw example", "btn raw load m": Value Change {
        # "load RAW command example"
        n101 = event-data() -> ()  [unwired: 1 in, 6 out]
        n102 = case shown="True" "btn raw load m" {
          frame False {
            # "load default as an example"
            n103 = invoke on="raw command" class="Str" method="Reinit To Default"() -> ()  [unwired: 3 in, 3 out]
          }
          frame True {
            # "load M-file"
            n104 = Read from Text File(prompt (Open existing file)="Select M-file to load") -> (text=w117:string, error out=w118:errorcluster)  [unwired: 3 in, 2 out]
            n105 = case shown="No Error" w118 {
              tunnel: w117 -> [w120 _]
              frame No Error {
                n106 = local write "raw command"(w120) -> ()
              }
              frame Error {
              }
            }
          }
        }
      }
      event "btn load algs": Value Change {
        # "this should also signalize\nalg. selector value change\nso algorithm view should update"
        # "Reload list of the QWTB algorithms"
        n107 = event-data() -> ()  [unwired: 1 in, 6 out]
        n108 = call "SGUI Set Control Enabled State By Groups.vi"("group name to enable (none)"="proc busy") -> ("error out"=w125:errorcluster)  [unwired: 9 in, 1 out]
        n109 = local read "session out"() -> (w127:T1)
        n110 = control-ref of="qwtb alg list"() -> (w128:refnum<vi>)
        n111 = call "Meas Proc QWTB Load List of Algorithms.vi"("menu ring ref"=w128, "error in"=w125, "session in"=w127) -> ("error out"=w123:errorcluster, "session out"=w126:T1)  [unwired: 6 in, 1 out]
        n112 = call "SGUI Set Control Enabled State By Groups.vi"("error in"=w123, "group name to enable (none)"="proc ready") -> ("error out"=w122:errorcluster)  [unwired: 8 in, 1 out]
        n113 = local write "session out"(w126) -> ()
        n114 = local write "error out"(w122) -> ()
      }
      event "qwtb alg list": Value Change {
        # "calc multi records visibility"
        # "update QWTB alg. view"
        n115 = event-data() -> ("OldVal"=w132:u16, "NewVal"=w131:u16)  [unwired: 1 in, 4 out]
        n116 = invoke on="qwtb var desc" class="Str" method="Reinit To Default"() -> ()  [unwired: 3 in, 3 out]
        n117 = Not Equal?(x=w132, y=w131) -> (x != y?=w130:bool)
        n118 = call "SGUI Set Control Enabled State By Groups.vi"("group name to enable (none)"="proc busy") -> ("error out"=w142:errorcluster)  [unwired: 9 in, 1 out]
        n119 = local read "session out"() -> (w153:T1)
        n120 = control-ref of="qwtb alg list"() -> (w129:refnum<vi>)
        n121 = control-ref of="qwtb unc mode"() -> (w137:refnum<vi>)
        n122 = control-ref of="qwtb alg params"() -> (w136:refnum<vi>)
        n123 = call "Meas Proc QWTB Load Algorithm.vi"("qwtb unc mode ref"=w137, "alg. selection changed?"=w130, "param table ref"=w136, "error in"=w142, "qwtb alg selector"=w129, "session in"=w153) -> ("error out"=w139:errorcluster, "qwtb alg flags"=w148:T68, "algorithm info"=w152:T69, "session out"=w135:T1)  [unwired: 1 in, 1 out]
        n124 = Unbundle By Name(w135) -> ("processing setup.QWTB.parsed parameters"=w134:T50[])
        n125 = Unbundle By Name(w152) -> ("description"=w150:string, "remark"=w151:string, "citation"=w149:string)
        n126 = local write "session out"(w135) -> ()
        n127 = Unbundle By Name(w148) -> ("supports differential transducer?"=w147:bool, "dual input algorithm?"=w146:bool, "supports multiple records?"=w145:bool)
        n128 = local write "qwtb alg desc"(w150) -> ()
        n129 = local write "qwtb alg note"(w151) -> ()
        n130 = local write "qwtb alg cite"(w149) -> ()
        n131 = local read "init parameters"() -> (w133:bool)
        n132 = case shown="True" w133 {
          selector: w133 -> [_ w156]
          tunnel: w139 -> [w154 w160]
          tunnel: [w154 w159] -> w138
          tunnel: w136 -> [_ w158]
          tunnel: w134 -> [_ w157]
          frame False {
          }
          frame True {
            n133 = Not(x=w156) -> (.not. x?=w155:bool)
            n134 = local write "init parameters"(w155) -> ()
            n135 = call "Meas Proc QWTB Set Params Table.vi"("error in"=w160, "qwtb parameters"=w157, "param table ref"=w158) -> ("error out"=w159:errorcluster)  [unwired: 8 in]
          }
        }
        n136 = call "SGUI Set Control Enabled State By Label.vi"("labels (empty)"="qwtb calc once", "Enabled? (False)"=w145) -> ()  [unwired: 8 in, 2 out]
        n137 = local write "qwtb alg is diff"(w147) -> ()
        n138 = local write "qwtb alg has ui"(w146) -> ()
        n139 = local write "qwtb calc once"(w145) -> ()
        n140 = call "SGUI Set Control Enabled State By Groups.vi"("error in"=w138, "group name to enable (none)"="proc ready") -> ("error out"=w140:errorcluster)  [unwired: 8 in, 1 out]
        n141 = local write "error out"(w140) -> ()
      }
      event "qwtb alg params": Mouse Up {
        # "update QWTB parameter info"
        n142 = event-data() -> ()  [unwired: 1 in, 8 out]
        n143 = call "SGUI Set Control Enabled State By Groups.vi"("group name to enable (none)"="proc busy") -> ("error out"=w164:errorcluster)  [unwired: 9 in, 1 out]
        n144 = local read "session out"() -> (w169:T1)
        n145 = control-ref of="qwtb alg params"() -> (w167:refnum<vi>)
        n146 = call "Meas Proc QWTB Get Input Parameter Info.vi"("param table ref"=w167, "error in"=w164, "session in"=w169) -> ("error out"=w162:errorcluster, "parameter description"=w166:string, "session out"=w168:T1)  [unwired: 6 in]
        n147 = local write "session out"(w168) -> ()
        n148 = local write "qwtb var desc"(w166) -> ()
        n149 = call "SGUI Set Control Enabled State By Groups.vi"("error in"=w162, "group name to enable (none)"="proc ready") -> ("error out"=w161:errorcluster)  [unwired: 8 in, 1 out]
        n150 = local write "error out"(w161) -> ()
      }
      event "btn qwtb clr params": Value Change {
        # "clear QWTB parameters table"
        n151 = event-data() -> ()  [unwired: 1 in, 6 out]
        n152 = invoke on="qwtb var desc" class="Str" method="Reinit To Default"() -> ()  [unwired: 3 in, 3 out]
        n153 = property on="qwtb alg params" class="Tbl (strict)"("Value"=string[][] [] ("qwtb alg params")) -> ()  [unwired: 2 in, 2 out]
      }
      event "btn mc cfg": Value Change {
        # "QWTB multicore setup"
        n154 = event-data() -> ()  [unwired: 1 in, 6 out]
        n155 = call "SGUI Set Control Enabled State By Groups.vi"("group name to enable (none)"="proc busy") -> ("error out"=w174:errorcluster)  [unwired: 9 in, 1 out]
        n156 = local read "session out"() -> (w177:T1)
        n157 = call "Meas Proc QWTB Multicore Panel.vi"("error in"=w174, "session in"=w177) -> ("error out"=w172:errorcluster, "session out"=w176:T1)  [unwired: 8 in]
        n158 = local write "session out"(w176) -> ()
        n159 = call "SGUI Set Control Enabled State By Groups.vi"("error in"=w172, "group name to enable (none)"="proc ready") -> ("error out"=w171:errorcluster)  [unwired: 8 in, 1 out]
        n160 = local write "error out"(w171) -> ()
      }
    }
  }
  n161 = flat-sequence {
    tunnel: w33 -> [_]
    tunnel: w25 -> [w181]
    tunnel: w16 -> [w178]
    frame #0 {
      w179 = SGUI_Assign_References_Mode."Release ID" ("register mode (overwrite)")
      # "on exit action - release GUI controls"
      n162 = call "SGUI Register Controls.vi"("register mode (overwrite)"=w179, "controls ID (empty)"=w181) -> ("error out"=w180:errorcluster)  [unwired: 15 in, 2 out]
      n163 = call "SGUI Register Controls Groups.vi"("error in"=w180, "register mode (overwrite)"=w179, "controls ID (empty)"=w178) -> ()  [unwired: 15 in, 2 out]
      n164 = call <vilib>:"Clear Errors.vi"() -> ()  [unwired: 7 in, 1 out]
    }
  }
